vi "ReCheckStrips.vi"(0 "Probe Card Channels":i32=32, 5 "Auto Re-Check":bool, 7 "Thresholds":T1, 9 "Bad channel list":i32[](array[numeric]), 10 "region in":u32, 11 "Number of strips probed":i32) -> (3 "Thresholds copy":T2 {"Hi R" format="%.2f"; "Lo R" format="%.2f"; "Current threshold" format="%.1f"; "Lo Cap" format="%.2f"; "Hi Cap" format="%.2f"})   [LabVIEW 2013]
uses:
  InstrControl/SupplyControl/SupplyControl.lvclass
  InstrControl/Switching/Switching.lvclass
  InstrControl/LCRControl/LCRControl.lvclass
  InstrControl/ProbeStationControl/ProbeStationControl.lvclass
  ProbePlan/ProbePlanParams.vi
  general_VIs/globals/QC_MeasurementSetup.vi
panel:
  out "Current Bias Voltage [V]":dbl
  out "Bias On/Off:":bool
  out "Single Needle":bool
  out "Strip Offset":i32
  in  "min scale array":i32[](array[numeric])
  in  "max scale array":i32[](array[numeric])
  out "Current [nA]":cluster{u32, i32, "Array OUT":dbl[]}(graph)
  out "Capacitance [pF]":cluster{u32, i32, "Array OUT":dbl[]}(graph)
  out "Resistance [MW]":cluster{u32, i32, "Array OUT":dbl[]}(graph)
  out "Region:":string
  out "Defects":string
  out "old R Data":dbl format="%.2f"
  out "Resistance":dbl format="%.2f"
  in  "go/stop":bool
  in  "Mode:":u16(ring) items=["Remeasure defect list", "Remeasure cursor strip"]
  in  "Edit Mode:":u16(ring) items=["Manual", "Automatic"]
  out "old flag":u16(ring) items=["Not known", "OK", "Pinhole", "Punchthrough", "Short", "Open", "Resistor", "Implant"]
  out "new flag":u16(ring) items=["Not yet known", "OK", "Pinhole", "Punchthrough", "Short", "Open", "Resistor", "Implant"]
  in  "Cursor Plot:":u16(ring) items=["Current", "Capacitance", "Resistance"]
  out "old C data":dbl format="%.2f"
  out "old I data":dbl format="%.2f"
  out "No. of strips checked":i32
  out "this strip no.":i32
  in  "update list":bool
  in  "Quit":bool
  out "Capacitance":dbl format="%.2f"
  out "Current":dbl format="%.2f"
  in  "skip this strip":bool
  in  "Correct Data":bool
  in  "Read":bool
  out "No. of bad channels":i32
  # "Analysis / Remeasurement of Strip Data"
  # "Current [nA]"
  # "Capacitance [pF]"
  # "Resistance [MW]"
  # "Thresholds"
  # "Measurements"
  # "Read / Edit Data"
  # "New Data                Old Data"
  # "No. checked:"
  # "Current:"
  # "Capacitance:"
  # "This Strip:"
  # "Resistance:"
  # "Defect?"
  # "Defect Channels"
  # "Number:"
  # "Current [nA]:"
  # "Capacitance [pF]:"
  # "Resistance [MW]:"
  # "Low              High"
  # "Current:"
  # "nA"
  # "Capacitance:"
  # "pF"
  # "Resistance:"
  # "Mohm"
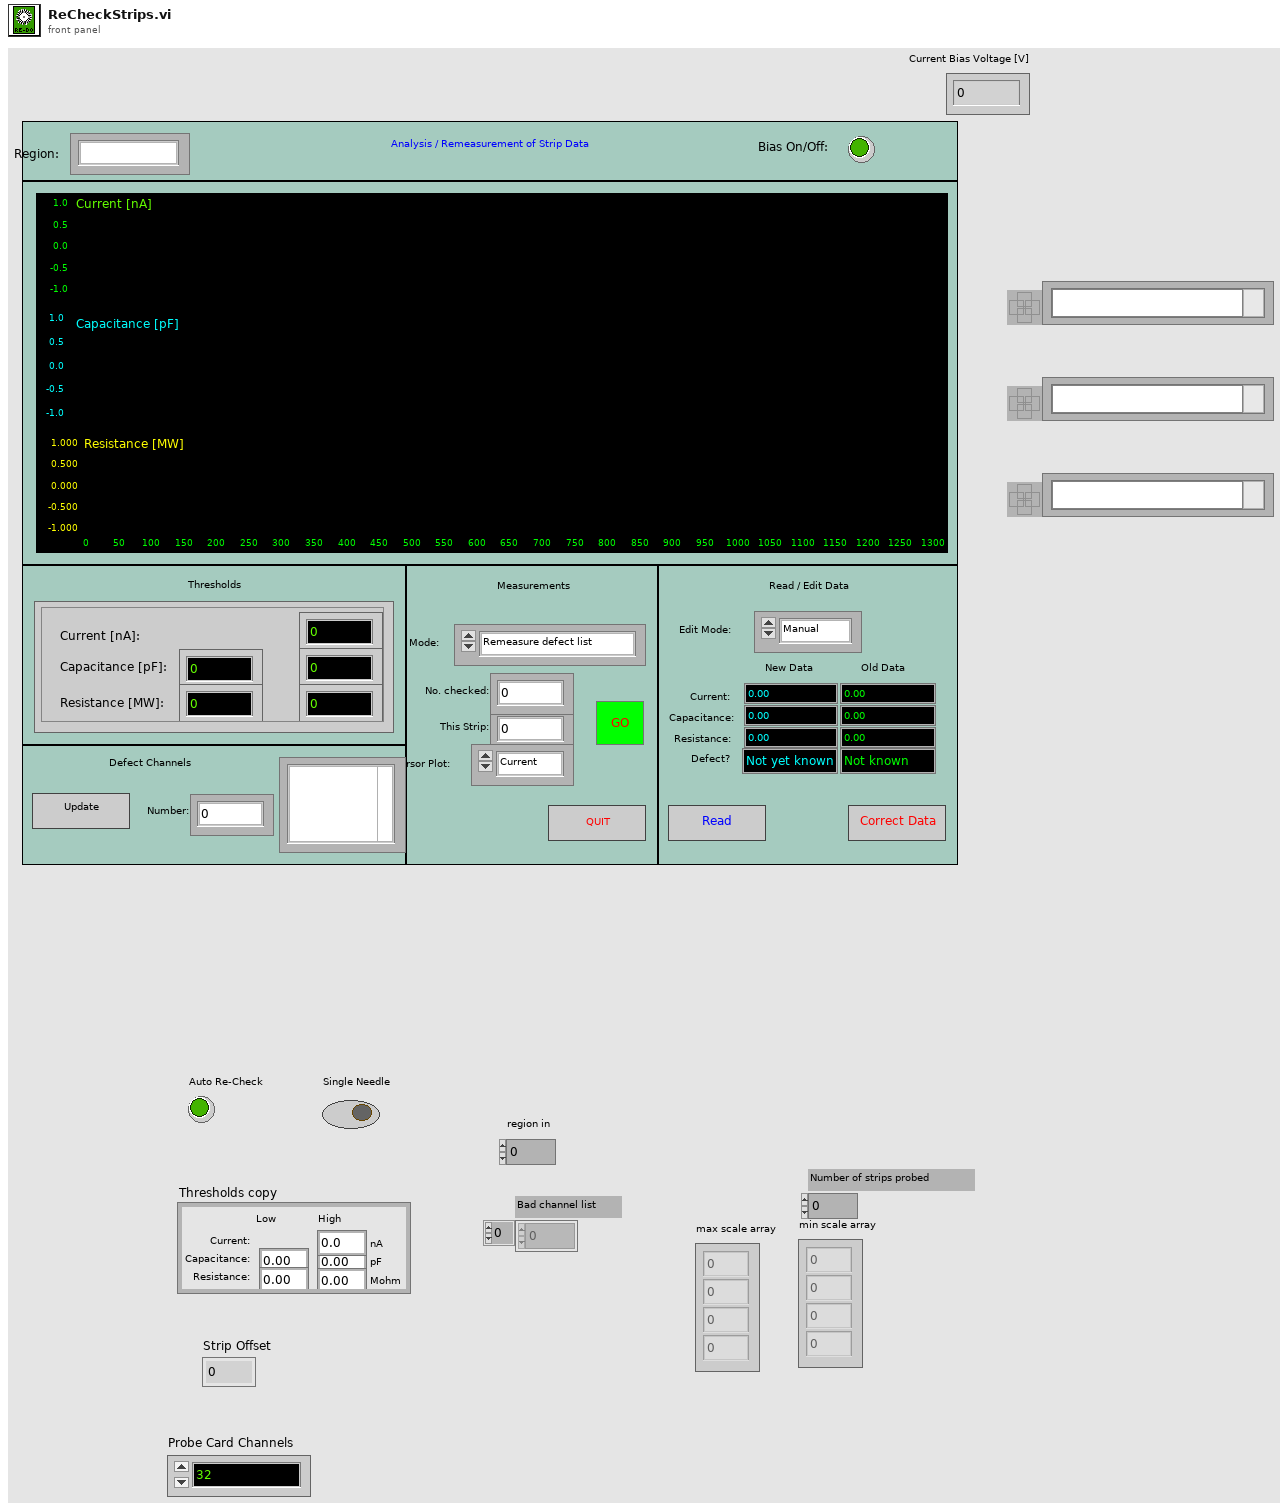
[diagram p1: front panel]
types:
  T1 = cluster{"Current [nA]":dbl, "Cap_Lo":dbl, "Cap_Hi":dbl, "Res_Hi":dbl, "Res_Lo":dbl}
  T2 = cluster{"Hi Cap":dbl, "Lo Cap":dbl, "Current threshold":dbl, "Lo R":dbl, "Hi R":dbl}
  T3 = cluster{"Strip Number OUT":i32, "X0":i32, "Y0":i32, "X1":i32, "Y1":i32, "Xref":dbl, "Yref":dbl, "ProbePlan type":u32, "Inner pads offset":ext, "Outer pads offset":ext, "l_inner":ext, "l_outer":ext, "strip numbering":u16, "Device Orientation":ext, "Stagger offset":i32, "Yoffset":dbl, "Strip pitch":dbl, "Fiducail separation":dbl, "Radius":ext, "Relative strip angles":dbl, "Probeplan description":string, "ProbePlan array":cluster{"Region":string, "ProbePoints":cluster{"X":dbl, "Y":dbl, "Label":string, "CardViable?":bool}[]}[], "Test ProbePoints":cluster{"Regions Enabled":bool[], "From index":u32[], "To index":u32[]}}
  T4 = cluster{"Region":string, "ProbePoints":cluster{"X":dbl, "Y":dbl, "Label":string, "CardViable?":bool}[]}[]
  T5 = cluster{"Region":string, "ProbePoints":cluster{"X":dbl, "Y":dbl, "Label":string, "CardViable?":bool}[]}
  T6 = enum16{"Reset", "Ground", "Striptest SMU", "Striptest LCR", "IV", "CV", "Interstrip Cap", "Interstrip Res"}
  T7 = cluster{"pass Rate in %":dbl, "Bad channel list":i32[], "No of bad strips":i32, "Defect description list":i32[], "Number of defects per category":i32[], "Defect lists":string[], "No of channels":i32, "Defect Flag array OUT":i32[][]}
  T8 = cluster{"Bias Supply":refnum<class "SupplyControl.lvclass">, "SMU":refnum<class "SupplyControl.lvclass">, "LCR":refnum<class "LCRControl.lvclass">, "Probe Card Channels":i32, "Bias Voltage [V]":dbl, "First strip":i32, "Last strip":i32, "Base Voltage [V]":dbl, "Base Ramp Step [V]":dbl, "Base Ramp Interval [ms]":u32, "High Voltage [V]":dbl, "High Ramp Step [V]":dbl, "High Ramp Interval [ms]":u32, "Single Needle":bool, "Temperature Readout":enum16{"Read Arduino", "Enter manually"}, "Arduino":refnum<class "ArduinoControl.lvclass">, "Fraction of good strips [%]":dbl, "ProbeStation":refnum<class "ProbeStationControl.lvclass">, "AC frequency [Hz]":i32, "Switching":refnum<class "Switching.lvclass">, "Matrix used?":bool, "Matrix X Channels":cluster{"Bias Supply / SMU LO":i32, "Bias Supply / SMU HI":i32, "CV Box LO":i32, "CV Box HI":i32, "CV Box LO IN":i32, "CV Box HI IN":i32, "Volt meter LO":i32, "Volt meter HI":i32, "Mux1 C1":i32, "Mux1 C2":i32, "Mux2 C1":i32, "Mux2 C2":i32}, "Pinholes Y/N":bool, "Capacitance Y/N":bool, "Resistance Y/N":bool}
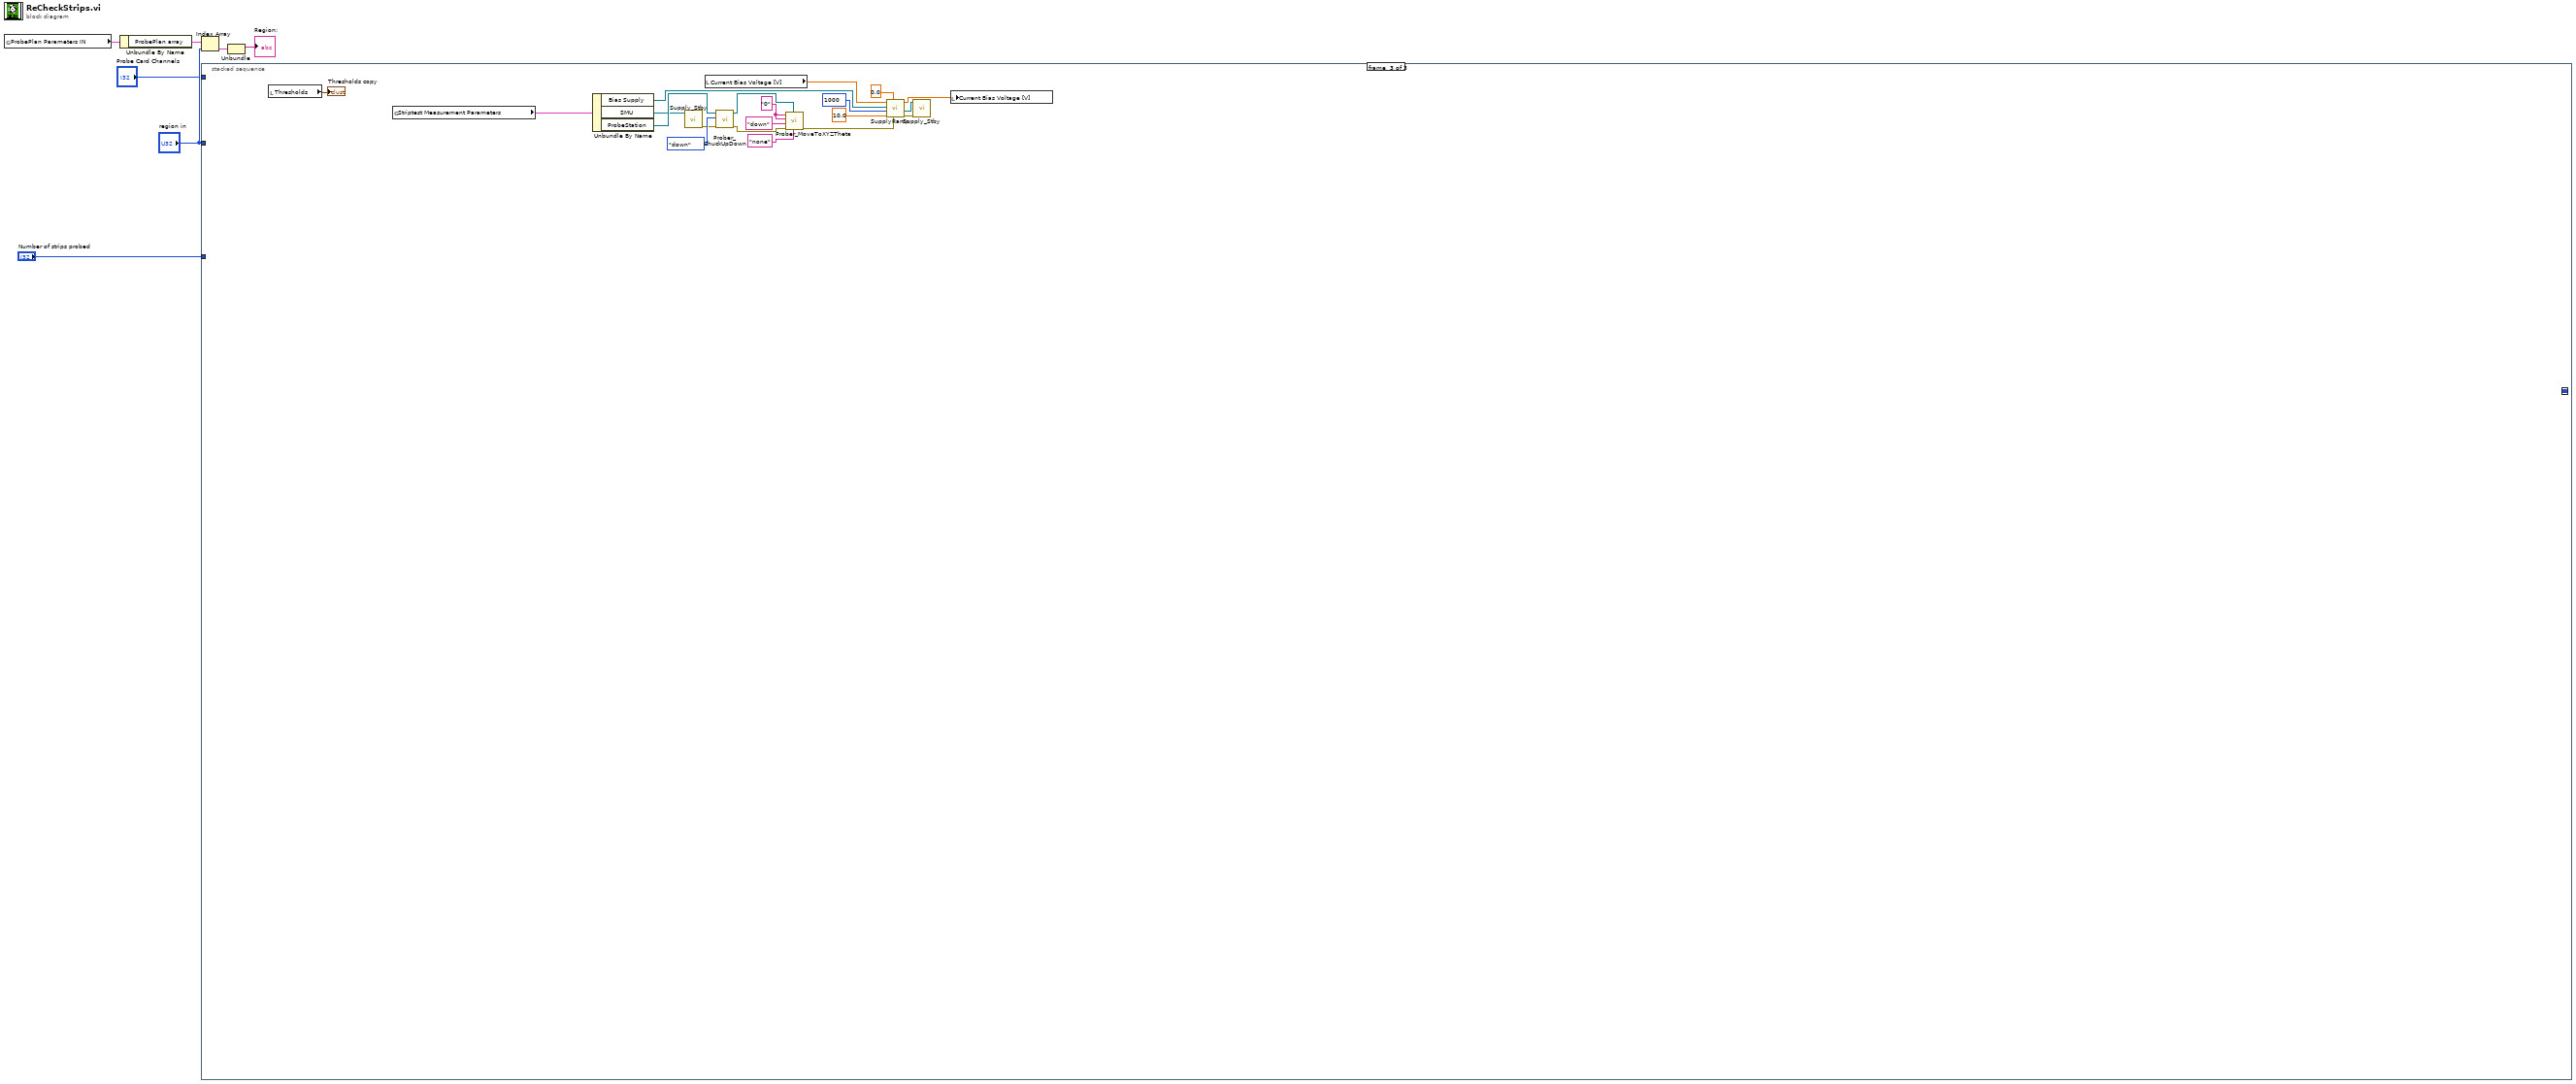
[diagram p0: block diagram]
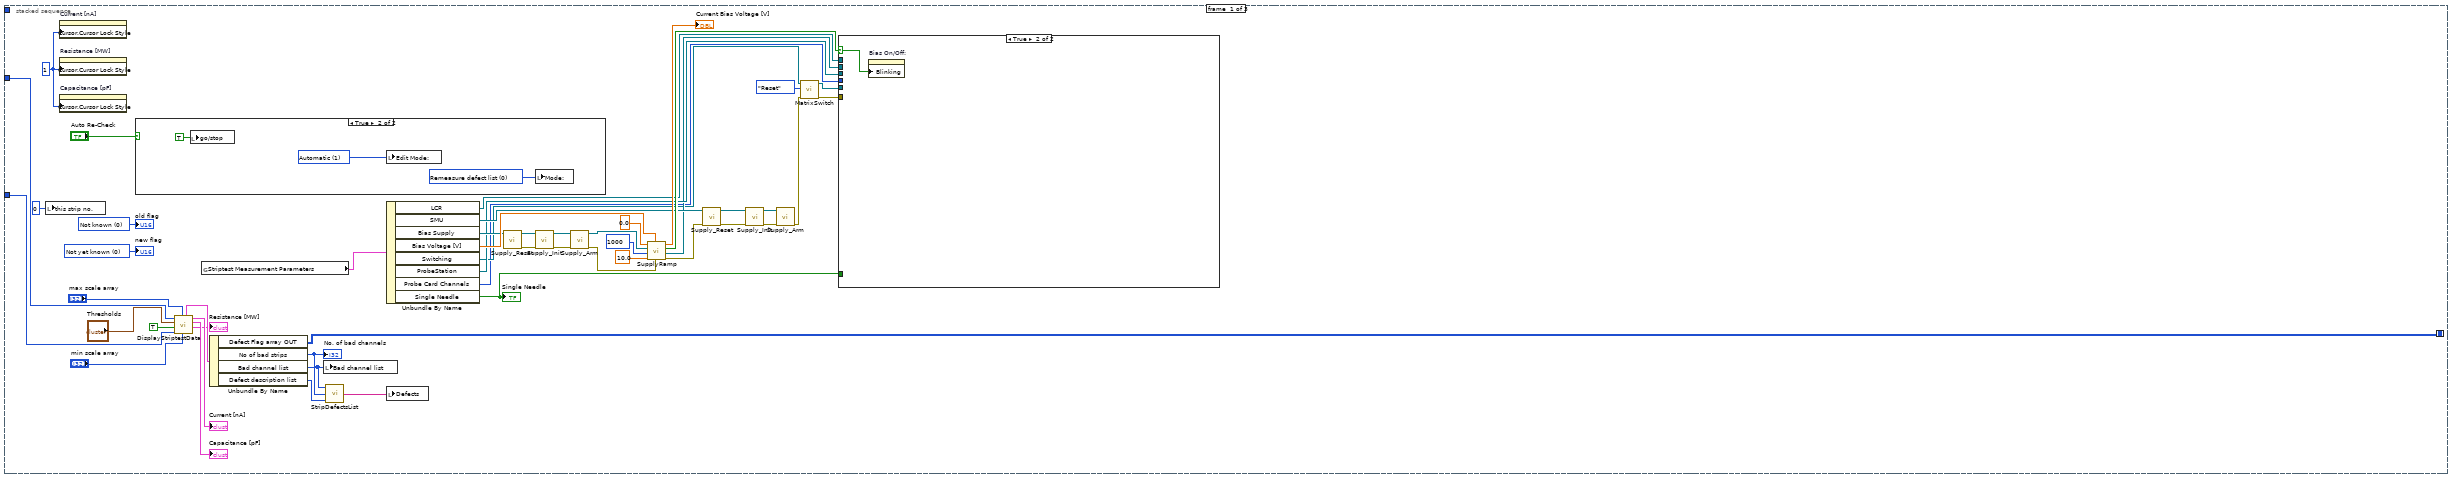
[diagram p2: hidden frame]
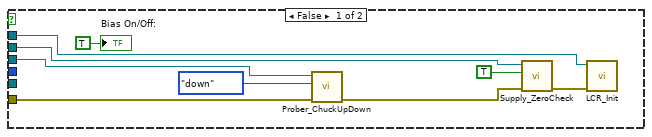
[diagram p3: hidden frame]
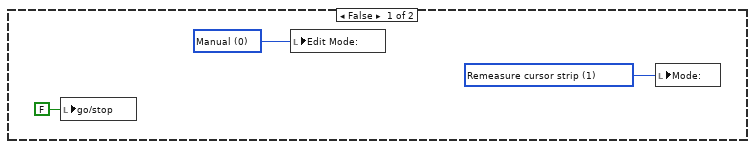
[diagram p4: hidden frame]
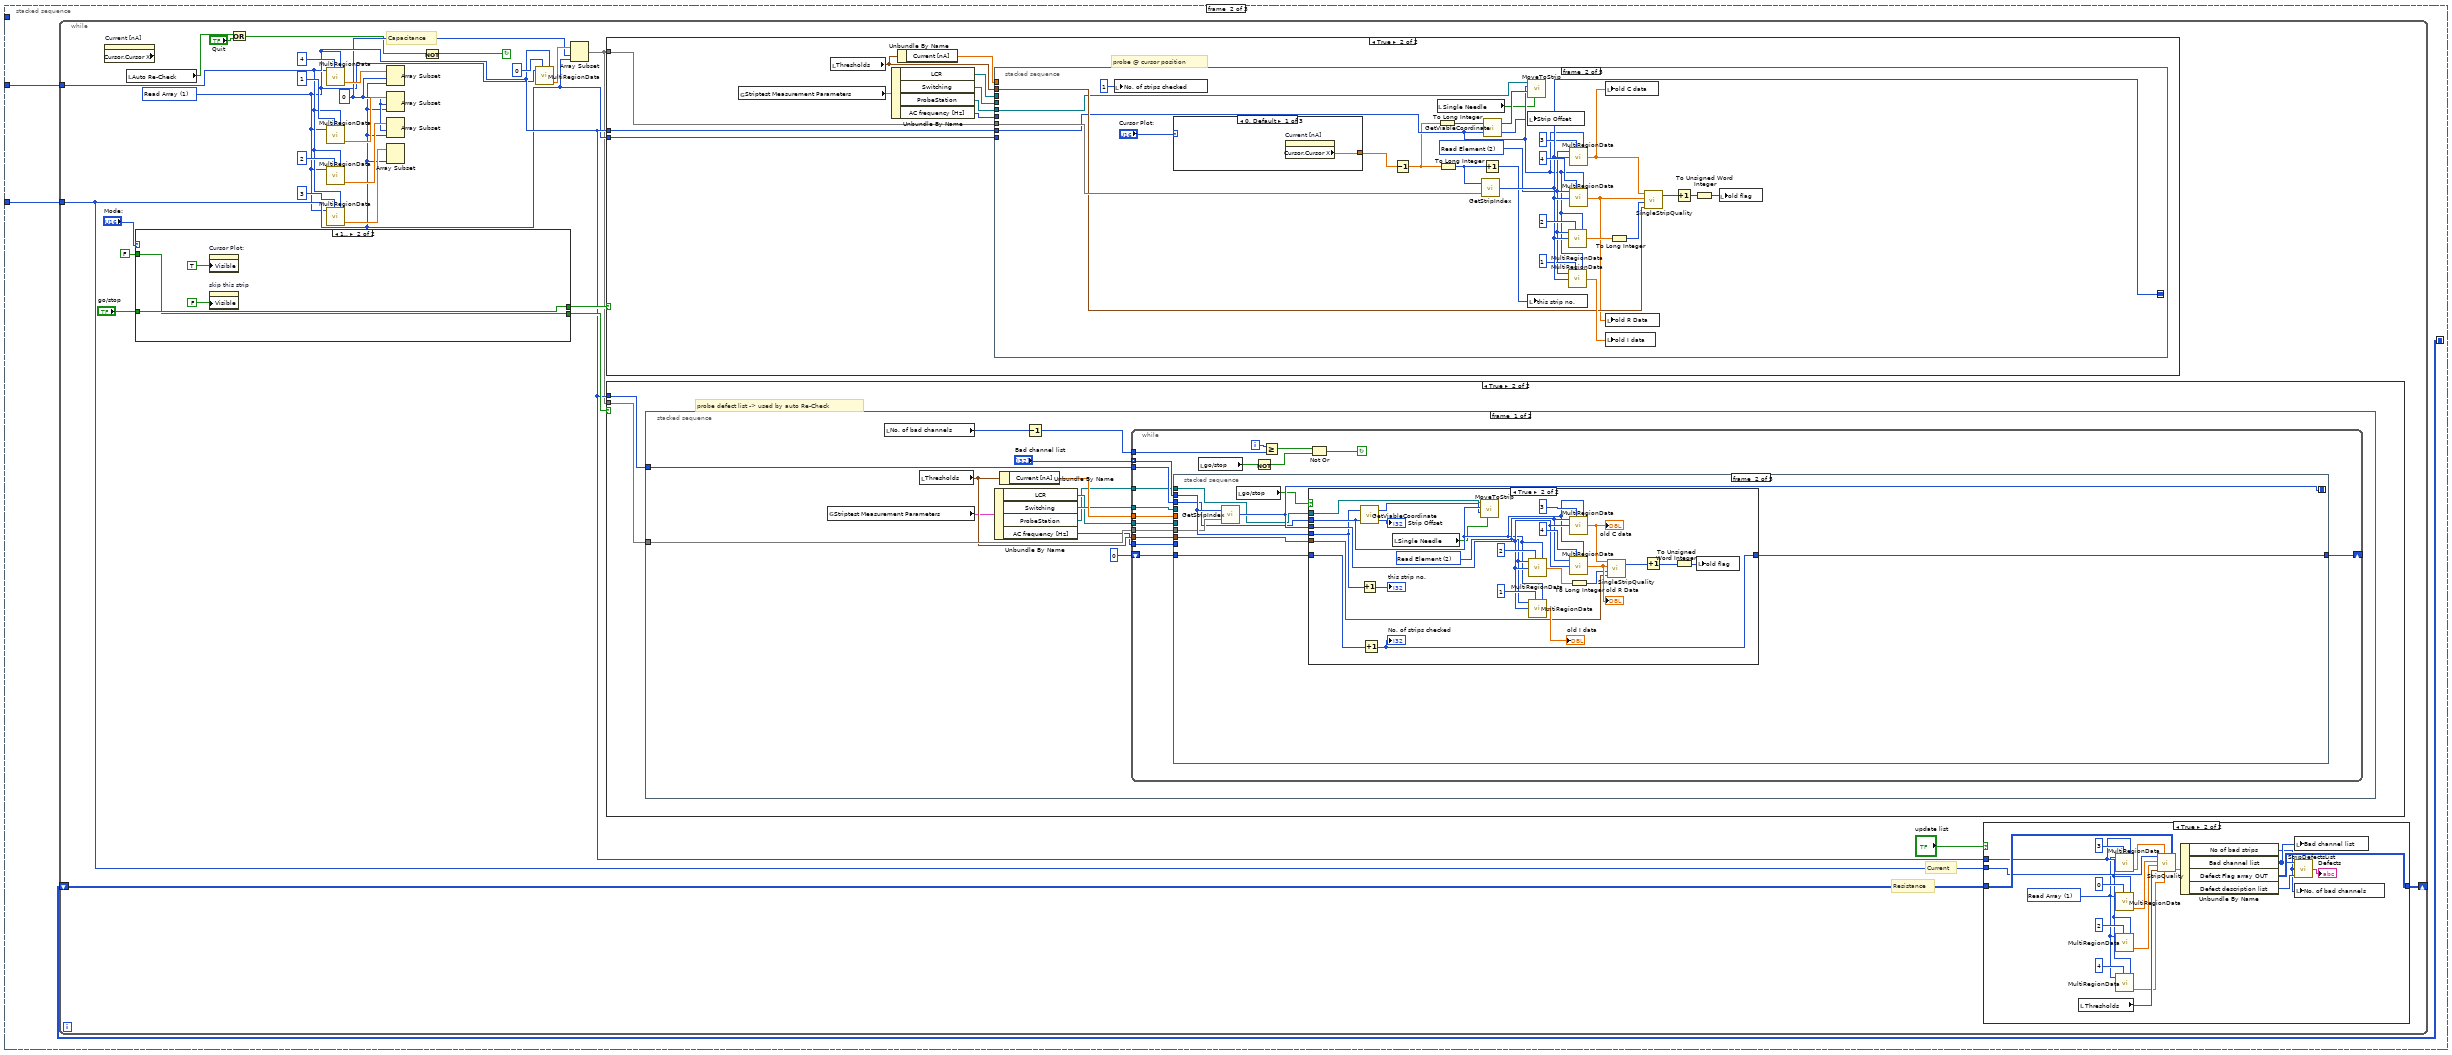
[diagram p5: hidden frame]
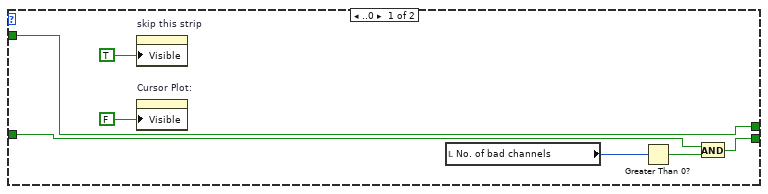
[diagram p6: hidden frame]
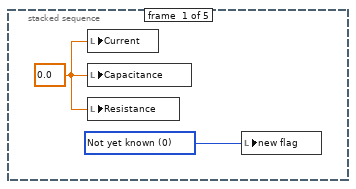
[diagram p8: hidden frame]
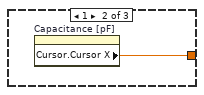
[diagram p9: hidden frame]
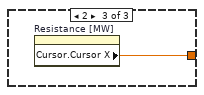
[diagram p10: hidden frame]
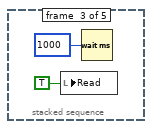
[diagram p11: hidden frame]
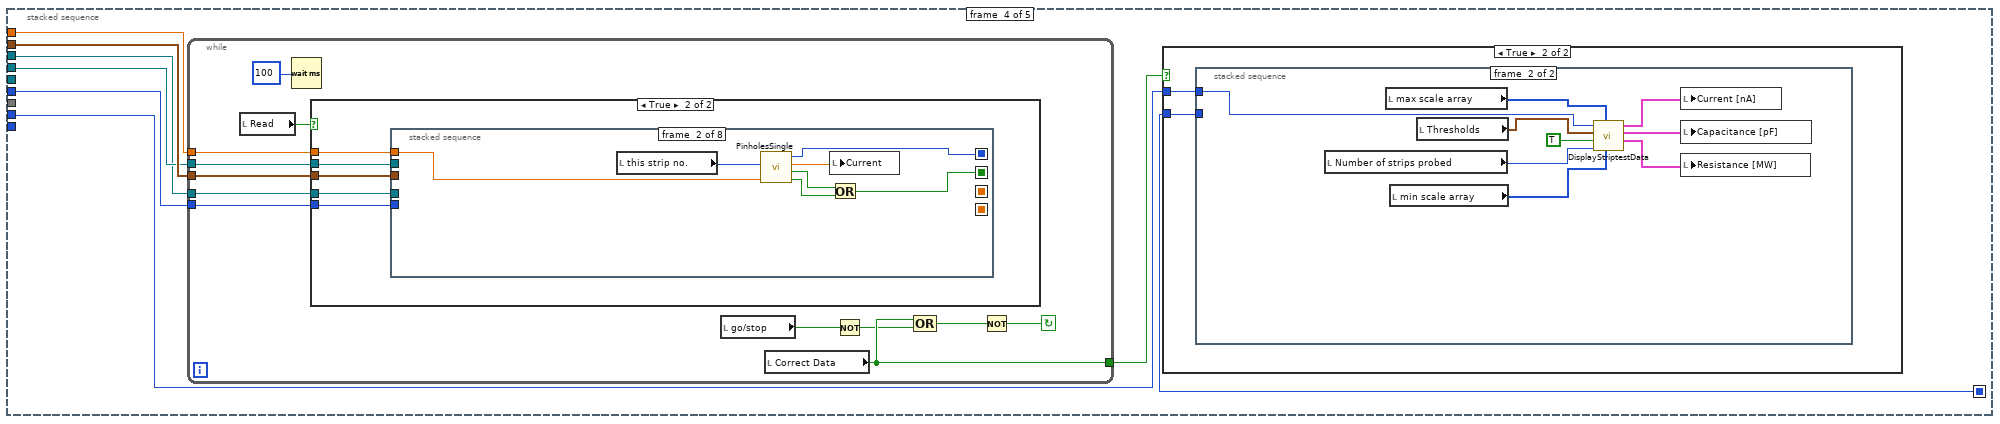
[diagram p12: hidden frame]
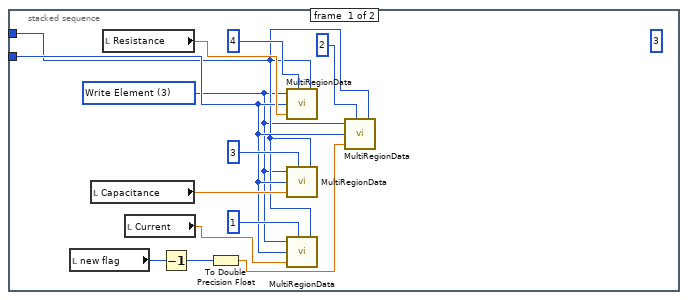
[diagram p14: hidden frame]
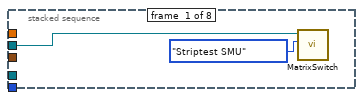
[diagram p16: hidden frame]
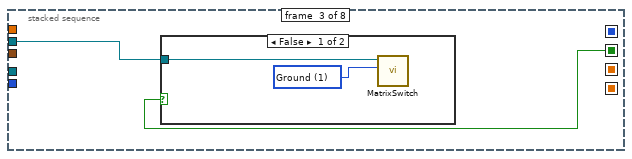
[diagram p17: hidden frame]
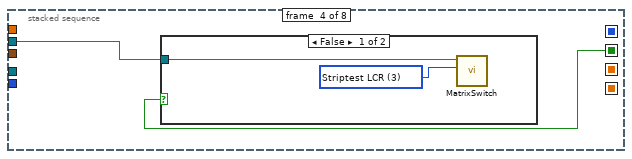
[diagram p19: hidden frame]
diagram:
  n1 = global read "ProbePlanParams.vi" "ProbePlan Parameters IN"() -> (w6:T3)
  n2 = Unbundle By Name(w6) -> ("ProbePlan array"=w5:T4)
  n3 = Index Array(array=w5, index="region in") -> (element=w3:T5)
  n4 = stacked-sequence {
    seq-local: [w56 _ _] -> [_ w74 _]
    tunnel: "Number of strips probed" -> [w46 w76 _]
    tunnel: "region in" -> [w48 w75 _]
    tunnel: "Probe Card Channels" -> [_ _ _]
    frame #0 {
      w53 = u16 0 items=["Not known", "OK", "Pinhole", "Punchthrough", "Short", "Open", "Resistor", "Implant"] ("old flag")
      w54 = u16 0 items=["Not yet known", "OK", "Pinhole", "Punchthrough", "Short", "Open", "Resistor", "Implant"] ("new flag")
      w42 = u32 1 ("Cursor Locked")
      n5 = local write "this strip no."(0 ("Current copy")) -> ()
      n6 = property on="Current [nA]" class="WFGraph (strict)"("Cursor.Cursor Lock Style"=w42) -> ()  [unwired: 2 in, 2 out]
      n7 = property on="Resistance [MW]" class="WFGraph (strict)"("Cursor.Cursor Lock Style"=w42) -> ()  [unwired: 2 in, 2 out]
      n8 = property on="Capacitance [pF]" class="WFGraph (strict)"("Cursor.Cursor Lock Style"=w42) -> ()  [unwired: 2 in, 2 out]
      n9 = case shown="True" "Auto Re-Check" {
        frame False {
          w68 = u16 0 items=["Manual", "Automatic"] ("Edit Mode:")
          w69 = u16 1 items=["Remeasure defect list", "Remeasure cursor strip"] ("Mode:")
          n10 = local write "go/stop"(FALSE ("Check strips")) -> ()
          n11 = local write "Edit Mode:"(w68) -> ()
          n12 = local write "Mode:"(w69) -> ()
        }
        frame True {
          w72 = u16 1 items=["Manual", "Automatic"] ("Edit Mode:")
          w73 = u16 0 items=["Remeasure defect list", "Remeasure cursor strip"] ("Mode:")
          n13 = local write "go/stop"(TRUE ("Check strips")) -> ()
          n14 = local write "Edit Mode:"(w72) -> ()
          n15 = local write "Mode:"(w73) -> ()
        }
      }
      n16 = call "DisplayStriptestData.vi"("min scale array"="min scale array", "max scale array"="max scale array", "# probed"=w46, "Display Stats?"=TRUE, "Thresholds"="Thresholds", "Region"=w48) -> ("Resistance [MW]"=→"Resistance [MW]":cluster{u32, i32, "Array OUT":dbl[]}, "Capacitance [pF]"=→"Capacitance [pF]":cluster{u32, i32, "Array OUT":dbl[]}, "Current [nA]"=→"Current [nA]":cluster{u32, i32, "Array OUT":dbl[]}, "Strip Quality Data"=w52:T7)  [unwired: 1 out]
      n17 = global read "QC_MeasurementSetup.vi" "Striptest Measurement Parameters"() -> (w8:T8)
      n18 = Unbundle By Name(w52) -> ("Defect Flag array OUT"=w56:i32[][], "No of bad strips"=w50:i32, "Bad channel list"=w49:i32[], "Defect description list"=w51:i32[])
      "No. of bad channels" <- w50
      n19 = local write "Bad channel list"(w49) -> ()
      n20 = call "StripDefectsList.vi"("Defect description list"=w51, "No of strips"=w50, "Bad channel list"=w49) -> ("Defect list"=w55:string)
      n21 = Unbundle By Name(w8) -> ("LCR"=w14:refnum<class "LCRControl.lvclass">, "SMU"=w15:refnum<class "SupplyControl.lvclass">, "Bias Supply"=w16:refnum<class "SupplyControl.lvclass">, "Bias Voltage [V]"=w26:dbl, "Switching"=w11:refnum<class "Switching.lvclass">, "ProbeStation"=w13:refnum<class "ProbeStationControl.lvclass">, "Probe Card Channels"=w10:i32, "Single Needle"=w9:bool)
      "Single Needle" <- w9
      n22 = local write "Defects"(w55) -> ()
      n23 = call-dynamic "Supply_Reset.vi"("SupplyControl in"=w16) -> ("error out"=w30:errorcluster, "SupplyControl out"=w33:refnum<class "SupplyControl.lvclass">)  [unwired: 9 in]
      n24 = call-dynamic "Supply_Init.vi"("error in (no error)"=w30, "SupplyControl in"=w33) -> ("error out"=w31:errorcluster, "SupplyControl out"=w32:refnum<class "SupplyControl.lvclass">)  [unwired: 8 in]
      n25 = call-dynamic "Supply_Arm.vi"("error in (no error)"=w31, "SupplyControl in"=w32) -> ("error out"=w28:errorcluster, "SupplyControl out"=w29:refnum<class "SupplyControl.lvclass">)  [unwired: 8 in]
      n26 = call "SupplyRamp.vi"("error in"=w28, "Requested Voltage"=w26, "Step Size"=10.0, "Step Delay"=1000, "Supply IN"=w29, "Starting Voltage"=0.0) -> ("error out"=w27:errorcluster, "Supply OUT"=w12:refnum<class "SupplyControl.lvclass">, "Compliance exceeded"=w20:bool, "Current Voltage"=→"Current Bias Voltage [V]":dbl)  [unwired: 2 in]
      n27 = call-dynamic "Supply_Reset.vi"("error in (no error)"=w27, "SupplyControl in"=w15) -> ("error out"=w24:errorcluster, "SupplyControl out"=w23:refnum<class "SupplyControl.lvclass">)  [unwired: 8 in]
      n28 = call-dynamic "Supply_Init.vi"("error in (no error)"=w24, "SupplyControl in"=w23) -> ("error out"=w25:errorcluster, "SupplyControl out"=w22:refnum<class "SupplyControl.lvclass">)  [unwired: 8 in]
      n29 = call-dynamic "Supply_Arm.vi"("error in (no error)"=w25, "SupplyControl in"=w22) -> ("error out"=w37:errorcluster)  [unwired: 8 in, 1 out]
      n30 = call-dynamic "MatrixSwitch.vi"("error in (no error)"=w37, "Action"=T6."Reset", "Switching in"=w11) -> ("error out"=w17:errorcluster, "Switching out"=w18:refnum<class "Switching.lvclass">)  [unwired: 6 in, 1 out]
      n31 = case shown="True" w20 {
        selector: w20 -> [_ w67]
        tunnel: w18 -> [_ _]
        tunnel: w17 -> [w66 _]
        tunnel: w14 -> [w63 _]
        tunnel: w13 -> [w65 _]
        tunnel: w12 -> [w62 _]
        tunnel: w10 -> [_ _]
        tunnel: w9 -> [_ _]
        frame False {
          n32 = call-dynamic "Prober_ChuckUpDown.vi"("error in (no error)"=w66, "Direction"=enum16{"up", "down"}."down", "ProbeStationControl in"=w65) -> ("error out"=w61:errorcluster)  [unwired: 6 in, 2 out]
          n33 = call-dynamic "Supply_ZeroCheck.vi"("error in (no error)"=w61, "enable/disable"=TRUE, "SupplyControl in"=w62) -> ("error out"=w58:errorcluster)  [unwired: 7 in, 1 out]
          n34 = call-dynamic "LCR_Init.vi"("error in (no error)"=w58, "LCRControl in"=w63) -> ()  [unwired: 8 in, 2 out]
          "Bias On/Off:" <- TRUE ("Bias On?")
        }
        frame True {
          n35 = property on="Bias On/Off:" class="Bool (strict)"("Blinking"=w67) -> ()  [unwired: 2 in, 2 out]
        }
      }
      "new flag" <- w54
      "old flag" <- w53
    }
    frame #1 {
      n36 = while {
        shift-right: [w98] -> _
        shift-left: w74 -> [w96]
        tunnel: w76 -> [w83]
        tunnel: w75 -> [w90]
        stop <- w103 continue-if-true
        w80 = u32 1 items=["Reset", "Read Array", "Read Element", "Write Element", "Write Array"] ("Action")
        w84 = 0
        # "Resistance"
        # "Capacitance"
        # "Current"
        n37 = property on="Current [nA]" class="WFGraph (strict)" props=["Cursor", "Cursor X"]() -> ()  [unwired: 2 in, 3 out]
        n38 = local read "Auto Re-Check"() -> (w79:bool)
        n39 = case shown="1.." "Mode:" {
          tunnel: "go/stop" -> [w108 w114]
          tunnel: [w107 w113] -> w101
          tunnel: [w106 w114] -> w100
          tunnel: FALSE -> [w106 w113]
          frame ..0 {
            n40 = property on="skip this strip" class="Bool"("Visible"=TRUE) -> ()  [unwired: 2 in, 2 out]
            n41 = property on="Cursor Plot:" class="Ring (strict)"("Visible"=FALSE) -> ()  [unwired: 2 in, 2 out]
            n42 = local read "No. of bad channels"() -> (w110:i32)
            n43 = Greater Than 0?(x=w110) -> (x > 0?=w109:bool)
            n44 = And(x=w108, y=w109) -> (x .and. y?=w107:bool)
          }
          frame 1.. {
            n45 = property on="Cursor Plot:" class="Ring (strict)"("Visible"=TRUE) -> ()  [unwired: 2 in, 2 out]
            n46 = property on="skip this strip" class="Bool"("Visible"=FALSE) -> ()  [unwired: 2 in, 2 out]
          }
        }
        n47 = Or(x=w79, y="Quit") -> (x .or. y?=w77:bool)
        n48 = call "MultiRegionData.vi"("Action"=w80, "Array No."=4, "Region index"=w90) -> ("Array OUT"=w88:dbl[])  [unwired: 3 in, 1 out]
        n49 = call "MultiRegionData.vi"("Action"=w80, "Array No."=1, "Region index"=w90) -> ("Array OUT"=w87:dbl[])  [unwired: 3 in, 1 out]
        n50 = call "MultiRegionData.vi"("Action"=w80, "Array No."=2, "Region index"=w90) -> ("Array OUT"=w86:dbl[])  [unwired: 3 in, 1 out]
        n51 = call "MultiRegionData.vi"("Action"=w80, "Array No."=3, "Region index"=w90) -> ("Array OUT"=w85:dbl[])  [unwired: 3 in, 1 out]
        n52 = Array Subset(array=w88, index=w84, length=w83) -> ()  [unwired: 1 out]
        n53 = Array Subset(array=w87, index=w84, length=w83) -> ()  [unwired: 1 out]
        n54 = Array Subset(array=w86, index=w84, length=w83) -> ()  [unwired: 1 out]
        n55 = Array Subset(array=w85, length=w83) -> ()  [unwired: 1 in, 1 out]
        n56 = Not(x=w77) -> (.not. x?=w103:bool)
        n57 = call "MultiRegionData.vi"("Action"=w80, "Array No."=0, "Region index"=w90) -> ("Array OUT"=w89:dbl[])  [unwired: 3 in, 1 out]
        n58 = Array Subset(array=w89, index=w84, length=w83) -> (w82:dbl[])
        n59 = case shown="True" w100 {
          tunnel: w82 -> [_ w124]
          tunnel: w83 -> [_ w121]
          tunnel: w90 -> [_ w120]
          frame False {
          }
          frame True {
            # "probe @ cursor position"
            n60 = global read "QC_MeasurementSetup.vi" "Striptest Measurement Parameters"() -> (w119:T8)
            n61 = local read "Thresholds"() -> (w122:T1)
            n62 = Unbundle By Name(w119) -> ("LCR"=w115:refnum<class "LCRControl.lvclass">, "Switching"=w117:refnum<class "Switching.lvclass">, "ProbeStation"=w118:refnum<class "ProbeStationControl.lvclass">, "AC frequency [Hz]"=w116:i32)
            n63 = Unbundle By Name(w122) -> ("Current [nA]"=w123:dbl)
            n64 = stacked-sequence {
              seq-local: [_ w148 _ _ _] -> [_ _ _ w166 _]
              tunnel: w124 -> [_ w151 _ _ _]
              tunnel: w123 -> [_ _ _ w165 _]
              tunnel: w122 -> [_ w143 _ w164 _]
              tunnel: w121 -> [_ _ _ _ _]
              tunnel: w120 -> [_ w134 _ w163 _]
              tunnel: w118 -> [_ w128 _ _ _]
              tunnel: w117 -> [_ _ _ w162 _]
              tunnel: w116 -> [_ _ _ w161 _]
              tunnel: w115 -> [_ _ _ w160 _]
              frame #0 {
                w125 = u16 0 items=["Not yet known", "OK", "Pinhole", "Punchthrough", "Short", "Open", "Resistor", "Implant"] ("new flag")
                w126 = 0.0 ("Current")
                n65 = local write "Current"(w126) -> ()
                n66 = local write "Capacitance"(w126) -> ()
                n67 = local write "Resistance"(w126) -> ()
                n68 = local write "new flag"(w125) -> ()
              }
              frame #1 {
                w137 = u32 2 items=["Reset", "Read Array", "Read Element", "Write Element", "Write Array"] ("Action")
                n69 = local write "No. of strips checked"(1 ("Current copy 2")) -> ()
                n70 = case shown="0, Default" "Cursor Plot:" {
                  tunnel: [w155 w156 w157] -> w132
                  frame 0, Default {
                    n71 = property on="Current [nA]" class="WFGraph (strict)"() -> ("Cursor.Cursor X"=w155:dbl)  [unwired: 2 in, 2 out]
                  }
                  frame 1 {
                    n72 = property on="Capacitance [pF]" class="WFGraph (strict)"() -> ("Cursor.Cursor X"=w156:dbl)  [unwired: 2 in, 2 out]
                  }
                  frame 2 {
                    n73 = property on="Resistance [MW]" class="WFGraph (strict)"() -> ("Cursor.Cursor X"=w157:dbl)  [unwired: 2 in, 2 out]
                  }
                }
                n74 = Decrement(x=w132) -> (x-1=w131:dbl)
                n75 = local read "Single Needle"() -> (w127:bool)
                n76 = To Long Integer(number=w131) -> (32bit integer=w135:i32)
                n77 = To Long Integer(number=w131) -> (32bit integer=w130:i32)
                n78 = call "GetStripIndex.vi"("Channel no array in"=w151, "Channel no. in"=w130) -> ("Index out"=w148:i32)
                n79 = call "GetViableCoordinate.vi"("Target Region [0-3]"=w134, "Actual Target Strip [0-1279]"=w135) -> ("Offset"=w133:i32, "Move Probecard to Strip #"=w136:i32)
                n80 = Increment(x=w130) -> (x+1=w129:i32)
                n81 = call "MoveToStrip.vi"("Single Needle"=w127, "Strip No."=w136, "Region"=w134, "ProbeStationControl in"=w128) -> ()  [unwired: 5 in, 3 out]
                n82 = local write "Strip Offset"(w133) -> ()
                n83 = local write "this strip no."(w129) -> ()
                n84 = call "MultiRegionData.vi"("Action"=w137, "Array No."=2, "Array Size / Index"=w148, "Region index"=w134) -> ("Data OUT"=w147:dbl)  [unwired: 2 in, 1 out]
                n85 = call "MultiRegionData.vi"("Action"=w137, "Array No."=1, "Array Size / Index"=w148, "Region index"=w134) -> ("Data OUT"=w154:dbl)  [unwired: 2 in, 1 out]
                n86 = call "MultiRegionData.vi"("Action"=w137, "Array No."=3, "Array Size / Index"=w148, "Region index"=w134) -> ("Data OUT"=w142:dbl)  [unwired: 2 in, 1 out]
                n87 = call "MultiRegionData.vi"("Action"=w137, "Array No."=4, "Array Size / Index"=w148, "Region index"=w134) -> ("Data OUT"=w141:dbl)  [unwired: 2 in, 1 out]
                n88 = local write "old C data"(w142) -> ()
                n89 = local write "old R Data"(w141) -> ()
                n90 = local write "old I data"(w154) -> ()
                n91 = To Long Integer(number=w147) -> (32bit integer=w146:i32)
                n92 = call "SingleStripQuality.vi"("Thresholds"=w143, "Pinhole flag in"=w146, "Resistance Data"=w141, "Capacitance Data"=w142) -> ("Defect Flag"=w140:i32)  [unwired: 2 in, 1 out]
                n93 = Increment(x=w140) -> (x+1=w139:i32)
                n94 = To Unsigned Word Integer(number=w139) -> (unsigned 16bit integer=w138:u16)
                n95 = local write "old flag"(w138) -> ()
              }
              frame #2 {
                n96 = local write "Read"(TRUE) -> ()
                n97 = Wait (ms)(milliseconds to wait=u32 1000 ("millisecond timer value")) -> ()  [unwired: 1 out]
              }
              frame #3 {
                n98 = while {
                  tunnel: [w199] -> w167
                  tunnel: w165 -> [w196]
                  tunnel: w164 -> [w195]
                  tunnel: w161 -> [w194]
                  tunnel: w162 -> [w193]
                  tunnel: w160 -> [w192]
                  stop <- w201 continue-if-true
                  n99 = local read "Read"() -> (w200:bool)
                  n100 = Wait (ms)(milliseconds to wait=100) -> ()  [unwired: 1 out]
                  n101 = case shown="True" w200 {
                    tunnel: w196 -> [_ w208]
                    tunnel: w195 -> [_ w207]
                    tunnel: w194 -> [_ w206]
                    tunnel: w193 -> [_ w205]
                    tunnel: w192 -> [_ w204]
                    frame False {
                    }
                    frame True {
                      n102 = stacked-sequence {
                        seq-local: [_ w216 _ _ _ _ _ _] -> [_ _ _ _ _ w243 _ _]
                        seq-local: [_ _ _ _ w230 _ _ _] -> [_ _ _ _ _ w242 _ _]
                        seq-local: [_ _ _ _ w229 _ _ _] -> [_ _ _ _ _ w241 _ _]
                        seq-local: [_ w212 _ _ _ _ _ _] -> [_ _ w219 w223 w227 _ _ _]
                        tunnel: w208 -> [_ w217 _ _ _ _ _ _]
                        tunnel: w207 -> [_ _ _ _ _ w240 _ _]
                        tunnel: w206 -> [_ _ _ _ w228 _ _ _]
                        tunnel: w205 -> [w209 _ w218 w222 _ _ _ _]
                        tunnel: w204 -> [_ _ _ _ w226 _ _ _]
                        frame #0 {
                          n103 = call-dynamic "MatrixSwitch.vi"("Action"=T6."Striptest SMU", "Switching in"=w209) -> ()  [unwired: 7 in, 3 out]
                        }
                        frame #1 {
                          n104 = local read "this strip no."() -> (w211:i32)
                          n105 = call "PinholesSingle.vi"("Current Threshold [nA]"=w217, "Channel"=w211) -> ("Compliance?"=w214:bool, "channel excluded"=w213:bool, "Current [nA]"=w215:dbl, "Flag"=w216:i32)  [unwired: 2 in]
                          n106 = local write "Current"(w215) -> ()
                          n107 = Or(x=w213, y=w214) -> (x .or. y?=w212:bool)
                        }
                        frame #2 {
                          n108 = case shown="False" w219 {
                            tunnel: w218 -> [w220 _]
                            frame False {
                              w221 = u16 1 items=["Reset", "Ground", "Striptest IV", "Striptest LCR", "IV", "CV", "Interstrip Cap", "Interstrip Res"] ("Action")
                              n109 = call-dynamic "MatrixSwitch.vi"("Action"=w221, "Switching in"=w220) -> ()  [unwired: 7 in, 3 out]
                            }
                            frame True {
                            }
                          }
                        }
                        frame #3 {
                          n110 = case shown="False" w223 {
                            tunnel: w222 -> [w224 _]
                            frame False {
                              w225 = u16 3 items=["Reset", "Ground", "Striptest IV", "Striptest LCR", "IV", "CV", "Interstrip Cap", "Interstrip Res"] ("Action")
                              n111 = call-dynamic "MatrixSwitch.vi"("Action"=w225, "Switching in"=w224) -> ()  [unwired: 7 in, 3 out]
                            }
                            frame True {
                            }
                          }
                        }
                        frame #4 {
                          n112 = case shown="True" w227 {
                            tunnel: [w231 w236] -> w230
                            tunnel: [w232 w235] -> w229
                            tunnel: w228 -> [_ w234]
                            tunnel: w226 -> [_ w233]
                            frame False {
                              n113 = local read "old R Data"() -> (w232:dbl)
                              n114 = local read "old C data"() -> (w231:dbl)
                            }
                            frame True {
                              n115 = call-dynamic "LCR_Readout.vi"("Frequency in Hz"=w234, "LCRControl in"=w233) -> ("Resistance in Ohm"=w235:dbl, "Capacitance in pF"=w236:dbl)  [unwired: 6 in, 2 out]
                              n116 = local write "Capacitance"(w236) -> ()
                              n117 = local write "Resistance"(w235) -> ()
                            }
                          }
                        }
                        frame #5 {
                          n118 = call "SingleStripQuality.vi"("Thresholds"=w240, "Pinhole flag in"=w243, "Resistance Data"=w241, "Capacitance Data"=w242) -> ("Defect Flag"=w239:i32)  [unwired: 2 in, 1 out]
                          n119 = Increment(x=w239) -> (x+1=w238:i32)
                          n120 = To Unsigned Word Integer(number=w238) -> (unsigned 16bit integer=w237:u16)
                          n121 = local write "new flag"(w237) -> ()
                        }
                        frame #6 {
                          n122 = local read "Edit Mode:"() -> (w245:u16)
                          n123 = Greater Than 0?(x=w245) -> (x > 0?=w244:bool)
                          n124 = local write "Correct Data"(w244) -> ()
                        }
                        frame #7 {
                          n125 = local write "Read"(FALSE ("Read")) -> ()
                        }
                      }
                    }
                  }
                  n126 = local read "go/stop"() -> (w198:bool)
                  n127 = local read "Correct Data"() -> (w199:bool)
                  n128 = Not(x=w198) -> (.not. x?=w197:bool)
                  n129 = Compound Arithmetic op=OR(w199, w197) -> (w202:bool)
                  n130 = Not(x=w202) -> (.not. x?=w201:bool)
                }
                n131 = case shown="True" w167 {
                  tunnel: w166 -> [_ w169]
                  tunnel: w163 -> [_ w168]
                  frame False {
                  }
                  frame True {
                    n132 = stacked-sequence {
                      tunnel: w169 -> [w172 _]
                      tunnel: w168 -> [w171 w188]
                      frame #0 {
                        w170 = u32 3 items=["Reset", "Read Array", "Read Element", "Write Element", "Write Array"] ("Action")
                        (unwired) u32 3 ("Action")
                        n133 = local read "new flag"() -> (w176:u16)
                        n134 = local read "Capacitance"() -> (w180:dbl)
                        n135 = local read "Resistance"() -> (w177:dbl)
                        n136 = local read "Current"() -> (w179:dbl)
                        n137 = Decrement(x=w176) -> (x-1=w174:u16)
                        n138 = To Double Precision Float(number=w174) -> (double precision float=w175:dbl)
                        n139 = call "MultiRegionData.vi"("Action"=w170, "Array No."=4, "Array Size / Index"=w172, "Data IN"=w177, "Region index"=w171) -> ()  [unwired: 1 in, 2 out]
                        n140 = call "MultiRegionData.vi"("Action"=w170, "Array No."=3, "Array Size / Index"=w172, "Data IN"=w180, "Region index"=w171) -> ()  [unwired: 1 in, 2 out]
                        n141 = call "MultiRegionData.vi"("Action"=w170, "Array No."=1, "Array Size / Index"=w172, "Data IN"=w179, "Region index"=w171) -> ()  [unwired: 1 in, 2 out]
                        n142 = call "MultiRegionData.vi"("Action"=w170, "Array No."=2, "Array Size / Index"=w172, "Data IN"=w175, "Region index"=w171) -> ()  [unwired: 1 in, 2 out]
                      }
                      frame #1 {
                        n143 = local read "Number of strips probed"() -> (w187:i32)
                        n144 = local read "max scale array"() -> (w183:i32[])
                        n145 = local read "min scale array"() -> (w184:i32[])
                        n146 = local read "Thresholds"() -> (w185:T1)
                        n147 = call "DisplayStriptestData.vi"("min scale array"=w184, "max scale array"=w183, "# probed"=w187, "Display Stats?"=TRUE, "Thresholds"=w185, "Region"=w188) -> ("Resistance [MW]"=w189:cluster{u32, i32, "Array OUT":dbl[]}, "Capacitance [pF]"=w190:cluster{u32, i32, "Array OUT":dbl[]}, "Current [nA]"=w191:cluster{u32, i32, "Array OUT":dbl[]})  [unwired: 2 out]
                        n148 = local write "Current [nA]"(w191) -> ()
                        n149 = local write "Capacitance [pF]"(w190) -> ()
                        n150 = local write "Resistance [MW]"(w189) -> ()
                      }
                    }
                  }
                }
              }
              frame #4 {
                w247 = FALSE
                n151 = local write "Read"(w247) -> ()
                n152 = local write "Correct Data"(w247) -> ()
                n153 = local write "go/stop"(w247) -> ()
              }
            }
          }
        }
        n154 = case shown="True" w101 {
          tunnel: w82 -> [_ w249]
          tunnel: w90 -> [_ w248]
          frame False {
          }
          frame True {
            # "probe defect list -> used by auto Re-Check"
            n155 = stacked-sequence {
              tunnel: w249 -> [w259 _]
              tunnel: w248 -> [w255 _]
              frame #0 {
                n156 = global read "QC_MeasurementSetup.vi" "Striptest Measurement Parameters"() -> (w254:T8)
                n157 = local read "No. of bad channels"() -> (w261:i32)
                n158 = local read "Thresholds"() -> (w256:T1)
                n159 = Unbundle By Name(w254) -> ("LCR"=w251:refnum<class "LCRControl.lvclass">, "Switching"=w253:refnum<class "Switching.lvclass">, "ProbeStation"=w250:refnum<class "ProbeStationControl.lvclass">, "AC frequency [Hz]"=w252:i32)
                n160 = Unbundle By Name(w256) -> ("Current [nA]"=w258:dbl)
                n161 = Decrement(x=w261) -> (x-1=w262:i32)
                n162 = while {
                  tunnel: "Bad channel list" -> [w268] mode=indexing
                  tunnel: w262 -> [w278]
                  shift-right: [w274] -> _
                  shift-left: 0 -> [w275]
                  tunnel: w258 -> [w273]
                  tunnel: w259 -> [w272]
                  tunnel: w256 -> [w269]
                  tunnel: w255 -> [w267]
                  tunnel: w253 -> [w266]
                  tunnel: w252 -> [w265]
                  tunnel: w251 -> [w264]
                  tunnel: w250 -> [w263]
                  i -> [w279]
                  stop <- w276 continue-if-true
                  n163 = stacked-sequence {
                    seq-local: [_ w287 _ _ _] -> [_ _ _ w326 _]
                    tunnel: w268 -> [_ w288 _ w322 _]
                    tunnel: w275 -> [_ w290 _ _ _]
                    tunnel: [_ w289 _ _ _] -> w274
                    tunnel: w273 -> [_ _ _ w325 _]
                    tunnel: w272 -> [_ w286 _ _ _]
                    tunnel: w269 -> [_ w284 _ w324 _]
                    tunnel: w267 -> [_ w283 _ w323 _]
                    tunnel: w266 -> [_ _ _ w321 _]
                    tunnel: w265 -> [_ _ _ w320 _]
                    tunnel: w264 -> [_ _ _ w319 _]
                    tunnel: w263 -> [_ w282 _ _ _]
                    frame #0 {
                      w280 = u16 0 items=["Not yet known", "OK", "Pinhole", "Punchthrough", "Short", "Open", "Resistor", "Implant"] ("new flag")
                      w281 = 0.0
                      n164 = local write "Current"(w281) -> ()
                      n165 = local write "Capacitance"(w281) -> ()
                      n166 = local write "Resistance"(w281) -> ()
                      n167 = local write "new flag"(w280) -> ()
                    }
                    frame #1 {
                      n168 = call "GetStripIndex.vi"("Channel no array in"=w286, "Channel no. in"=w288) -> ("Index out"=w287:i32)
                      n169 = local read "go/stop"() -> (w285:bool)
                      n170 = case shown="True" w285 {
                        tunnel: [w291 w315] -> w289
                        tunnel: w290 -> [w291 w314]
                        tunnel: w288 -> [_ w295]
                        tunnel: w287 -> [_ w300]
                        tunnel: w284 -> [_ w304]
                        tunnel: w283 -> [_ w298]
                        tunnel: w282 -> [_ w292]
                        frame False {
                        }
                        frame True {
                          w299 = u32 2 items=["Reset", "Read Array", "Read Element", "Write Element", "Write Array"] ("Action")
                          n171 = call "GetViableCoordinate.vi"("Target Region [0-3]"=w298, "Actual Target Strip [0-1279]"=w295) -> ("Offset"=→"Strip Offset":i32, "Move Probecard to Strip #"=w297:i32)
                          n172 = Increment(x=w295) -> (x+1=→"this strip no.":i32)
                          n173 = Increment(x=w314) -> (x+1=w315:i32)
                          "No. of strips checked" <- w315
                          n174 = local read "Single Needle"() -> (w293:bool)
                          n175 = call "MoveToStrip.vi"("Single Needle"=w293, "Strip No."=w297, "Region"=w298, "ProbeStationControl in"=w292) -> ()  [unwired: 5 in, 3 out]
                          n176 = call "MultiRegionData.vi"("Action"=w299, "Array No."=2, "Array Size / Index"=w300, "Region index"=w298) -> ("Data OUT"=w306:dbl)  [unwired: 2 in, 1 out]
                          n177 = call "MultiRegionData.vi"("Action"=w299, "Array No."=1, "Array Size / Index"=w300, "Region index"=w298) -> ("Data OUT"=→"old I data":dbl)  [unwired: 2 in, 1 out]
                          n178 = call "MultiRegionData.vi"("Action"=w299, "Array No."=3, "Array Size / Index"=w300, "Region index"=w298) -> ("Data OUT"=w308:dbl)  [unwired: 2 in, 1 out]
                          "old C data" <- w308
                          n179 = call "MultiRegionData.vi"("Action"=w299, "Array No."=4, "Array Size / Index"=w300, "Region index"=w298) -> ("Data OUT"=w307:dbl)  [unwired: 2 in, 1 out]
                          "old R Data" <- w307
                          n180 = To Long Integer(number=w306) -> (32bit integer=w305:i32)
                          n181 = call "SingleStripQuality.vi"("Thresholds"=w304, "Pinhole flag in"=w305, "Resistance Data"=w307, "Capacitance Data"=w308) -> ("Defect Flag"=w303:i32)  [unwired: 2 in, 1 out]
                          n182 = Increment(x=w303) -> (x+1=w302:i32)
                          n183 = To Unsigned Word Integer(number=w302) -> (unsigned 16bit integer=w301:u16)
                          n184 = local write "old flag"(w301) -> ()
                        }
                      }
                    }
                    frame #2 {
                      n185 = local read "go/stop"() -> (w316:bool)
                      n186 = case shown="True" w316 {
                        frame False {
                        }
                        frame True {
                          n187 = local write "Read"(TRUE ("Read")) -> ()
                          n188 = Wait (ms)(milliseconds to wait=u32 1000) -> ()  [unwired: 1 out]
                        }
                      }
                    }
                    frame #3 {
                      n189 = while {
                        tunnel: ["Correct Data"] -> w327
                        tunnel: w325 -> [w359]
                        tunnel: w324 -> [w356]
                        tunnel: w322 -> [w355]
                        tunnel: w321 -> [w354]
                        tunnel: w320 -> [w353]
                        tunnel: w319 -> [w352]
                        stop <- w360 continue-if-true
                        n190 = Wait (ms)(milliseconds to wait=u32 100) -> ()  [unwired: 1 out]
                        n191 = case shown="True" "Read" {
                          tunnel: w359 -> [_ w371]
                          tunnel: w356 -> [_ w370]
                          tunnel: w355 -> [_ w369]
                          tunnel: w354 -> [_ w368]
                          tunnel: w353 -> [_ w367]
                          tunnel: w352 -> [_ w366]
                          frame False {
                          }
                          frame True {
                            n192 = stacked-sequence {
                              seq-local: [_ w379 _ _ _ _ _ _] -> [_ _ _ _ _ w406 _ _]
                              seq-local: [_ _ _ _ w393 _ _ _] -> [_ _ _ _ _ w405 _ _]
                              seq-local: [_ _ _ _ w392 _ _ _] -> [_ _ _ _ _ w404 _ _]
                              seq-local: [_ w375 _ _ _ _ _ _] -> [_ _ w382 w386 w390 _ _ _]
                              tunnel: w371 -> [_ w380 _ _ _ _ _ _]
                              tunnel: w370 -> [_ _ _ _ _ w403 _ _]
                              tunnel: w367 -> [_ _ _ _ w391 _ _ _]
                              tunnel: w369 -> [_ w374 _ _ _ _ _ _]
                              tunnel: w368 -> [w372 _ w381 w385 _ _ _ _]
                              tunnel: w366 -> [_ _ _ _ w389 _ _ _]
                              frame #0 {
                                w373 = u16 2 items=["Reset", "Ground", "Striptest IV", "Striptest LCR", "IV", "CV", "Interstrip Cap", "Interstrip Res"] ("Action")
                                n193 = call-dynamic "MatrixSwitch.vi"("Action"=w373, "Switching in"=w372) -> ()  [unwired: 7 in, 3 out]
                              }
                              frame #1 {
                                n194 = call "PinholesSingle.vi"("Current Threshold [nA]"=w380, "Channel"=w374) -> ("Compliance?"=w376:bool, "channel excluded"=w377:bool, "Current [nA]"=→"Current":dbl, "Flag"=w379:i32)  [unwired: 2 in]
                                n195 = Or(x=w377, y=w376) -> (x .or. y?=w375:bool)
                              }
                              frame #2 {
                                n196 = case shown="False" w382 {
                                tunnel: w381 -> [w383 _]
                                frame False {
                                w384 = u16 1 items=["Reset", "Ground", "Striptest IV", "Striptest LCR", "IV", "CV", "Interstrip Cap", "Interstrip Res"] ("Action")
                                n197 = call-dynamic "MatrixSwitch.vi"("Action"=w384, "Switching in"=w383) -> ()  [unwired: 7 in, 3 out]
                                }
                                frame True {
                                }
                                }
                              }
                              frame #3 {
                                n198 = case shown="False" w386 {
                                tunnel: w385 -> [w387 _]
                                frame False {
                                w388 = u16 3 items=["Reset", "Ground", "Striptest IV", "Striptest LCR", "IV", "CV", "Interstrip Cap", "Interstrip Res"] ("Action")
                                n199 = call-dynamic "MatrixSwitch.vi"("Action"=w388, "Switching in"=w387) -> ()  [unwired: 7 in, 3 out]
                                }
                                frame True {
                                }
                                }
                              }
                              frame #4 {
                                n200 = case shown="False" w390 {
                                tunnel: [w397 w398] -> w393
                                tunnel: [w396 w399] -> w392
                                tunnel: w391 -> [w395 _]
                                tunnel: w389 -> [w394 _]
                                frame False {
                                n201 = call-dynamic "LCR_Readout.vi"("Frequency in Hz"=w395, "LCRControl in"=w394) -> ("Resistance in Ohm"=w396:dbl, "Capacitance in pF"=w397:dbl)  [unwired: 6 in, 2 out]
                                "Capacitance" <- w397
                                "Resistance" <- w396
                                }
                                frame True {
                                n202 = local read "old R Data"() -> (w399:dbl)
                                n203 = local read "old C data"() -> (w398:dbl)
                                }
                                }
                              }
                              frame #5 {
                                n204 = call "SingleStripQuality.vi"("Thresholds"=w403, "Pinhole flag in"=w406, "Resistance Data"=w404, "Capacitance Data"=w405) -> ("Defect Flag"=w402:i32)  [unwired: 2 in, 1 out]
                                n205 = Increment(x=w402) -> (x+1=w401:i32)
                                n206 = To Unsigned Word Integer(number=w401) -> (unsigned 16bit integer=w400:u16)
                                n207 = local write "new flag"(w400) -> ()
                              }
                              frame #6 {
                                n208 = Greater Than 0?(x="Edit Mode:") -> (x > 0?=w407:bool)
                                n209 = local write "Correct Data"(w407) -> ()
                              }
                              frame #7 {
                                n210 = local write "Read"(FALSE ("Read")) -> ()
                              }
                            }
                          }
                        }
                        n211 = local read "go/stop"() -> (w358:bool)
                        n212 = Not(x=w358) -> (.not. x?=w357:bool)
                        n213 = Compound Arithmetic op=OR("Correct Data", "skip this strip", w357) -> (w361:bool)
                        n214 = Not(x=w361) -> (.not. x?=w360:bool)
                      }
                      n215 = case shown="True" w327 {
                        tunnel: w326 -> [_ w329]
                        tunnel: w323 -> [_ w328]
                        frame False {
                        }
                        frame True {
                          n216 = stacked-sequence {
                            tunnel: w329 -> [w332 _]
                            tunnel: w328 -> [w331 w343]
                            frame #0 {
                              w330 = u32 3 items=["Reset", "Read Array", "Read Element", "Write Element", "Write Array"] ("Action")
                              n217 = local read "new flag"() -> (w335:u16)
                              n218 = local read "Capacitance"() -> (w341:dbl)
                              n219 = local read "Resistance"() -> (w337:dbl)
                              n220 = local read "Current"() -> (w342:dbl)
                              n221 = Decrement(x=w335) -> (x-1=w334:u16)
                              n222 = To Double Precision Float(number=w334) -> (double precision float=w333:dbl)
                              n223 = call "MultiRegionData.vi"("Action"=w330, "Array No."=3, "Array Size / Index"=w332, "Data IN"=w341, "Region index"=w331) -> ()  [unwired: 1 in, 2 out]
                              n224 = call "MultiRegionData.vi"("Action"=w330, "Array No."=1, "Array Size / Index"=w332, "Data IN"=w342, "Region index"=w331) -> ()  [unwired: 1 in, 2 out]
                              n225 = call "MultiRegionData.vi"("Action"=w330, "Array No."=4, "Array Size / Index"=w332, "Data IN"=w337, "Region index"=w331) -> ()  [unwired: 1 in, 2 out]
                              n226 = call "MultiRegionData.vi"("Action"=w330, "Array No."=2, "Array Size / Index"=w332, "Data IN"=w333, "Region index"=w331) -> ()  [unwired: 1 in, 2 out]
                            }
                            frame #1 {
                              n227 = local read "Number of strips probed"() -> (w347:i32)
                              n228 = local read "max scale array"() -> (w351:i32[])
                              n229 = local read "min scale array"() -> (w350:i32[])
                              n230 = local read "Thresholds"() -> (w349:T1)
                              n231 = call "DisplayStriptestData.vi"("min scale array"=w350, "max scale array"=w351, "# probed"=w347, "Display Stats?"=TRUE, "Thresholds"=w349, "Region"=w343) -> ("Resistance [MW]"=w346:cluster{u32, i32, "Array OUT":dbl[]}, "Capacitance [pF]"=w345:cluster{u32, i32, "Array OUT":dbl[]}, "Current [nA]"=w344:cluster{u32, i32, "Array OUT":dbl[]})  [unwired: 2 out]
                              n232 = local write "Current [nA]"(w344) -> ()
                              n233 = local write "Capacitance [pF]"(w345) -> ()
                              n234 = local write "Resistance [MW]"(w346) -> ()
                            }
                          }
                        }
                      }
                    }
                    frame #4 {
                      w410 = FALSE
                      n235 = local write "Read"(w410) -> ()
                      n236 = local write "Correct Data"(w410) -> ()
                    }
                  }
                  n237 = local read "go/stop"() -> (w271:bool)
                  n238 = Not(x=w271) -> (.not. x?=w270:bool)
                  n239 = Greater Or Equal?(x=w279, y=w278) -> (x >= y?=w277:bool)
                  n240 = Not Or(1:w270, 2:w277) -> (0:w276:bool)
                }
              }
              frame #1 {
                w411 = FALSE ("Read")
                n241 = local write "go/stop"(FALSE ("Check strips")) -> ()
                n242 = local write "Read"(w411) -> ()
                n243 = local write "Correct Data"(w411) -> ()
              }
            }
          }
        }
        n244 = case shown="True" "update list" {
          tunnel: w96 -> [w413 w432]
          tunnel: w83 -> [_ w425]
          tunnel: [w413 w426] -> w98
          tunnel: w90 -> [_ w415]
          frame False {
          }
          frame True {
            w414 = u32 1 items=["Reset", "Read Array", "Read Element", "Write Element", "Write Array"] ("Action")
            n245 = local read "Thresholds"() -> (w421:T1)
            n246 = call "MultiRegionData.vi"("Action"=w414, "Array No."=3, "Region index"=w415) -> ("Array OUT"=w417:dbl[])  [unwired: 3 in, 1 out]
            n247 = call "MultiRegionData.vi"("Action"=w414, "Array No."=0, "Region index"=w415) -> ("Array OUT"=w416:dbl[])  [unwired: 3 in, 1 out]
            n248 = call "MultiRegionData.vi"("Action"=w414, "Array No."=2, "Region index"=w415) -> ("Array OUT"=w418:dbl[])  [unwired: 3 in, 1 out]
            n249 = call "MultiRegionData.vi"("Action"=w414, "Array No."=4, "Region index"=w415) -> ("Array OUT"=w419:dbl[])  [unwired: 3 in, 1 out]
            n250 = call "StripQuality.vi"("No of entries"=w425, "Capacitance Data Array"=w417, "Channel No. Array"=w416, "Pinhole flag array in"=w418, "Resistance data array"=w419, "Thresholds"=w421, "Defect Flag array IN"=w432) -> ("Strip Quality Data"=w427:T7)  [unwired: 1 out]
            n251 = Unbundle By Name(w427) -> ("No of bad strips"=w420:i32, "Bad channel list"=w423:i32[], "Defect Flag array OUT"=w426:i32[][], "Defect description list"=w424:i32[])
            n252 = local write "Bad channel list"(w423) -> ()
            n253 = call "StripDefectsList.vi"("Defect description list"=w424, "No of strips"=w420, "Bad channel list"=w423) -> ("Defect list"=→"Defects":string)
            n254 = local write "No. of bad channels"(w420) -> ()
          }
        }
      }
    }
    frame #2 {
      w450 = "0"
      n255 = local read "Thresholds"() -> (→"Thresholds copy":T1)
      n256 = global read "QC_MeasurementSetup.vi" "Striptest Measurement Parameters"() -> (w439:T8)
      n257 = Unbundle By Name(w439) -> ("Bias Supply"=w437:refnum<class "SupplyControl.lvclass">, "SMU"=w434:refnum<class "SupplyControl.lvclass">, "ProbeStation"=w438:refnum<class "ProbeStationControl.lvclass">)
      n258 = call-dynamic "Supply_Stby.vi"("SupplyControl in"=w434) -> ("error out"=w433:errorcluster)  [unwired: 9 in, 1 out]
      n259 = local read "Current Bias Voltage [V]"() -> (w443:dbl)
      n260 = call-dynamic "Prober_ChuckUpDown.vi"("error in (no error)"=w433, "Direction"=enum16{"up", "down"}."down", "ProbeStationControl in"=w438) -> ("error out"=w446:errorcluster, "ProbeStationControl out"=w445:refnum<class "ProbeStationControl.lvclass">)  [unwired: 6 in, 1 out]
      n261 = call-dynamic "Prober_MoveToXYZTheta.vi"("Theta location [mdeg]"="none", "ProbeStationControl in"=w445, "error in (no error)"=w446, "Z location [µm]"="down", "Y location [µm]"=w450, "X location [µm]"=w450) -> ("error out"=w444:errorcluster)  [unwired: 3 in, 2 out]
      n262 = call "SupplyRamp.vi"("error in"=w444, "Requested Voltage"=0.0, "Step Size"=10.0, "Step Delay"=1000, "Supply IN"=w437, "Starting Voltage"=w443) -> ("error out"=w436:errorcluster, "Supply OUT"=w435:refnum<class "SupplyControl.lvclass">, "Current Voltage"=w442:dbl)  [unwired: 2 in, 1 out]
      n263 = call-dynamic "Supply_Stby.vi"("error in (no error)"=w436, "SupplyControl in"=w435) -> ()  [unwired: 8 in, 2 out]
      n264 = local write "Current Bias Voltage [V]"(w442) -> ()
    }
  }
  n265 = Unbundle(w3) -> ("Region"=→"Region:":string)  [unwired: 1 out]
